vi "DSF.Engine.Plugin.Iteration.Increment.vi"(8 "error in (no error)":errorcluster, 11 "Plugin in":refnum<class "DSF.Engine.Plugin.lvclass">) -> (0 "error out":errorcluster, 3 "Plugin out":refnum<class "DSF.Engine.Plugin.lvclass">)   [LabVIEW 2017, in "DSF.Engine.lvlib" / "DSF.Engine.Plugin.lvclass"]
uses:
  DSF.Engine.Plugin.lvclass
  DSF.Engine.Plugin.lvclass/DSF.Engine.Plugin.ctl
  Timing/DSF.Engine.Timing.lvclass/DSF.Engine.Timing.ctl
  Timing/DSF.Engine.Timing.Get Iteration.vi
  Timing/DSF.Engine.Timing.Set Iteration.vi
  Timing/DSF.Engine.Timing.lvclass
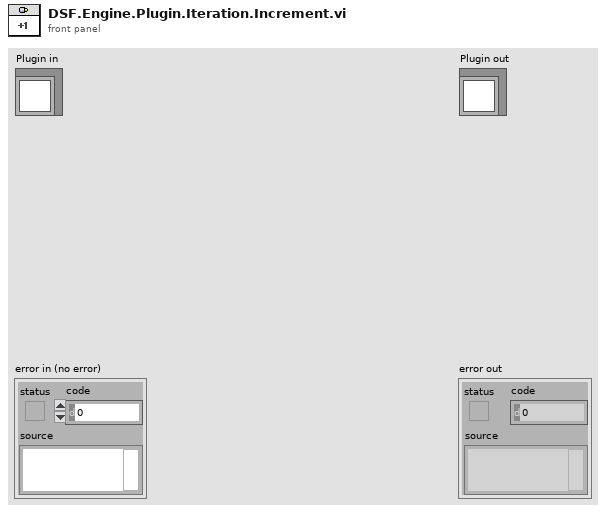
[diagram p1: front panel]
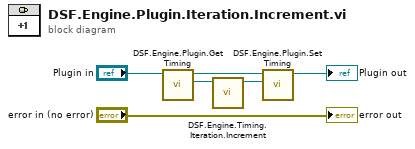
[diagram p0: block diagram]
diagram:
  n1 = call "DSF.Engine.Plugin.Get Timing.vi"("Plugin in"="Plugin in") -> ("Timing"=w5:refnum<class "DSF.Engine.Timing.lvclass">, "Plugin out"=w3:refnum<class "DSF.Engine.Plugin.lvclass">)  [unwired: 9 in]
  n2 = call "DSF.Engine.Timing.Iteration.Increment.vi"("Timing in"=w5) -> ("Timing out"=w4:refnum<class "DSF.Engine.Timing.lvclass">)  [unwired: 10 in]
  n3 = call "DSF.Engine.Plugin.Set Timing.vi"("Timing"=w4, "Plugin in"=w3) -> ("Plugin out"=→"Plugin out":refnum<class "DSF.Engine.Plugin.lvclass">)  [unwired: 9 in]
  "error out" <- "error in (no error)"
